vi "SVFA FFT Spectrum (Mag-Phase) (N Ch).vi"(0 "scaled signals [EU]":waveform(dbl)[](array[waveform]), 2 "window":T8=1 items=["None"=0, "Hanning"=1, "Hamming"=2, "Blackman-Harris"=3, "Exact Blackman"=4, "Blackman"=5, "Flat Top"=6, "4 Term B-Harris "=7, "7 Term B-Harris"=8, "Low Sidelobe"=9, "Force"=64, "Exponential"=65, "Blackman Nuttall"=11, "Triangle"=30, "Bartlett-Hanning"=31, "Bohman"=32, "Parzen"=33, "Welch"=34, "Kaiser"=60, "Dolph-Chebyshev"=61, "Gaussian"=62], 4 "view":T9={"dB On (T)"=TRUE, "unwrap phase (F)"=FALSE, "convert to degree (T)"=TRUE}, 5 "error in (no error)":errorcluster, 7 "averaging parameters":T7={"averaging mode"=enum."No averaging", "weighting mode"=enum."Exponential", "number of averages"=10, "linear mode"=enum."One shot"} {"number of averages" min=1 step=1}, 9 "restart averaging (F)":bool) -> (11 "averaging done":bool, 13 "averages completed":dbl, 14 "magnitudes [dB EU]":cluster{"f0":dbl, "df":dbl, "magnitude":dbl[]}[](array[cluster]) {"magnitude" format="%.2p"; "df" format="%.2p"; "f0" format="%.2p"}, 15 "magnitude unit labels":string[](array[string]), 16 "phases [degrees]":cluster{"f0":dbl, "df":dbl, "phase":dbl[]}[](array[cluster]) {"phase" format="%.2f"; "df" format="%.2f"; "f0" format="%.2f"}, 17 "phase unit labels":string[](array[string]), 18 "spectrum info":T1[](array[typedef]) {"x-axis units" items=["Time (s)"=0, "Frequency-CB (Hz)"=1, "Frequency-CPB (Hz)"=1248, "Frequency-Arbitrary (Hz)"=2357, "Quefrency (s)"=2, "Revolutions (rev)"=3, "Order"=4, "Speed (RPM)"=11, "Speed (rad/s)"=21, "Index"=65535]; "weighting filter" items=["Linear", "A-weighting", "B-weighting", "C-weighting", "ITU-R 468-4", "Dolby", "CCITT", "C-message", "Wb", "Wc", "Wd", "We", "Wf", "Wh", "Wj", "Wk", "Wm", "AES17 20 kHz lowpass", "AES17 40 kHz lowpass", "AES17 20 kHz highpass", "AES17 40 kHz highpass"]; "dB reference [EU]" format="%.2f"; "engineering units" items=["custom..."=0, "V"=1, "A"=21, "C"=30, "pC"=31, "s"=32, "-"=29, "Pa"=2, "N"=20, "g"=3, "m/s^2"=4, "m/s"=5, "m"=6, "mm/s"=12, "mm"=13, "micron/s"=14, "micron"=15, "in/s^2"=7, "in/s"=8, "in"=9, "mil/s"=10, "mil"=11, "rad/s^2"=16, "rad/s"=17, "rad"=18, "deg/s^2"=26, "deg/s"=27, "deg"=28, "RPM"=22, "cycle/s^2"=23, "Hz"=24, "cycle"=25, "strain"=19]; "spectral info"."window" items=["None "=0, "Hanning"=1, "Hamming"=2, "Blackman-Harris"=3, "Exact Blackman"=4, "Blackman"=5, "Flat Top"=6, "4 Term B-Harris "=7, "7 Term B-Harris"=8, "Low Sidelobe"=9, "Force - Exponential"=10, "Gaussian"=62]}, 19 "error out":errorcluster)   [LabVIEW 2017]
doc: "Computes the Fast Fourier Transform (FFT) spectrum of <B>scaled signal [EU]</B>. This VI returns FFT results as the magnitude and phase of the FFT spectrum. Wire data to the <B>scaled signal [EU]</B> input to determine the polymorphic instance to use or manually select the instance."
uses:
  <vilib>/addons/_NISVFA/_Shared subVIs/Controls/svc_Window.ctl
  <vilib>/addons/_NISVFA/_Shared subVIs/Controls/svc_Spectrum Info.ctl
  <vilib>/addons/_NISVFA/_Shared subVIs/Controls/svc_X-Axis Units.ctl
  <vilib>/addons/_NISVFA/_Shared subVIs/Controls/svc_Spectrum Type.ctl
  <vilib>/addons/_NISVFA/_Shared subVIs/Controls/svc_Engineering Units Text Ring.ctl
  <vilib>/addons/_NISVFA/_Shared subVIs/Controls/svc_Weighting Filter Text Ring.ctl
  <vilib>/addons/_NISVFA/_Shared subVIs/Controls/svc_Complimentary Spectrum Units.ctl
  <vilib>/Analysis/2dsp.llb/Real FFT.vi
  <vilib>/Analysis/2dsp.llb/Power Spectrum (DBL).vi
  <vilib>/addons/_NISVFA/_Shared subVIs/Windowing/svfa_Scaled Time Domain Window (1 Ch).vi
  <vilib>/addons/_NISVFA/_Shared subVIs/Spectrum Info/svfa_Build Spectrum Info.vi
  <vilib>/addons/_NISVFA/_Shared subVIs/Spectrum Averaging/svfa_No Average Array (complex).vi
  <vilib>/addons/_NISVFA/_Shared subVIs/Spectrum Averaging/svfa_Average Array (complex).vi
  <vilib>/addons/_NISVFA/_Shared subVIs/Spectrum Averaging/svfa_No Average Array (real).vi
  <vilib>/addons/_NISVFA/_Shared subVIs/Spectrum Averaging/svfa_Average Array (real).vi
  <vilib>/addons/_NISVFA/_Shared subVIs/Spectrum Averaging/svfa_Peak Hold Array.vi
  <vilib>/addons/_NISVFA/_Shared subVIs/Windowing/svfa_Scaled Time Domain Window (Array).vi
  <vilib>/addons/_NISVFA/_Shared subVIs/Common/svc_Get SV Channel Info.vi
  <vilib>/addons/_NISVFA/_Shared subVIs/Common/svc_Spectrum Units.vi
  <vilib>/Analysis/4window.llb/Force Window.vi
  <vilib>/Analysis/4window.llb/Force Window (DBL).vi
  <vilib>/Analysis/4window.llb/Exponential Window.vi
  <vilib>/Analysis/4window.llb/Exponential Window (DBL).vi
  <vilib>/Utility/error.llb/Error Cluster From Error Code.vi
  <vilib>/Analysis/0measdsp.llb/Scaled Time Domain Window.vi
  <vilib>/Analysis/0measdsp.llb/Scaled Time Domain Window (DBL).vi
  <vilib>/addons/_NISVFA/_Spectrum Processing/subVIs/svfa_Spectrum Info Window to windowTd Type Def.vi
  <vilib>/addons/_NISVFA/_Shared subVIs/Common/svc_Window Parameters.vi
  <vilib>/addons/_NISVFA/_Shared subVIs/Common/svc_Get Window Info.vi
  <vilib>/addons/_NISVFA/_Shared subVIs/Common/svc_Get Weighting Enum and Labels.vi
  <vilib>/addons/_NISVFA/_Shared subVIs/Common/svc_Unit Label Lexical Class.vi
  <vilib>/addons/_NISVFA/_Shared subVIs/Common/svc_Engineering Units to Unit Label.vi
  <vilib>/addons/_NISVFA/_Shared subVIs/Common/svc_Format Value (DBL).vi
  <vilib>/addons/_NISVFA/_Shared subVIs/Common/svc_Channel Info to Spectrum Info.vi
  <vilib>/addons/_NISVFA/_Shared subVIs/Common/svc_Unit Label to Engineering Units.vi
  <vilib>/Analysis/NI_AALPro.lvlib
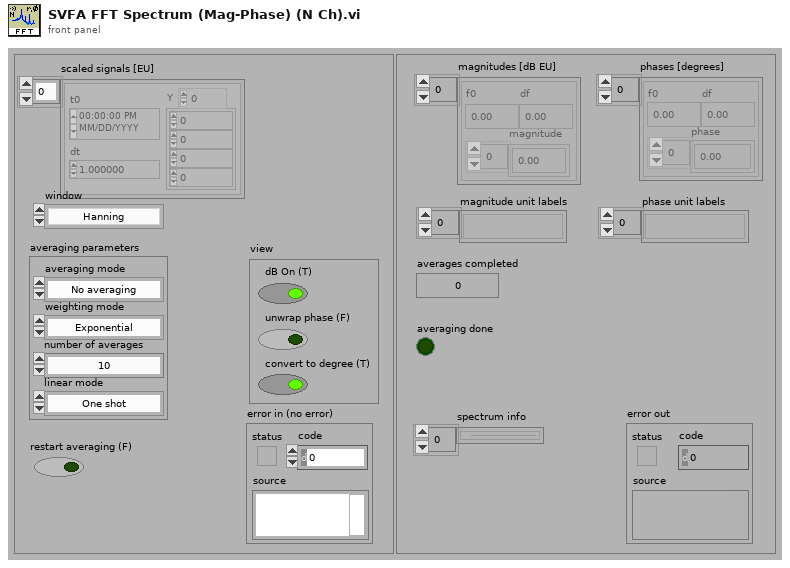
[diagram p1: front panel]
types:
  T1 = typedef "svc_Spectrum Info.ctl" = cluster{"channel name":string, "description":string, "x-axis units":T2, "spectral info":cluster{"spectrum type":T3, "linear/dB":enum16{"linear", "dB"}, "window":u16, "window size":i32, "FFT size":i32}, "engineering units":T4, "custom label":string, "dB reference [EU]":dbl, "peak units":enum16{"rms", "peak", "peak-peak"}, "weighting filter":T5, "spectral density?":bool, "unit label":string, "spectrum skewed?":bool, "complimentary spectrum units":T6}
  T2 = typedef "svc_X-Axis Units.ctl" = u16
  T3 = typedef "svc_Spectrum Type.ctl" = enum16{"FFT Spectrum [complex]", "Amplitude [Magnitude]", "Power [Magnitude^2]", "Cross Spectrum [complex]", "Frequency Response [Complex]"}
  T4 = typedef "svc_Engineering Units Text Ring.ctl" = u16
  T5 = typedef "svc_Weighting Filter Text Ring.ctl" = u16
  T6 = typedef "svc_Complimentary Spectrum Units.ctl" = enum16{"none", "radians", "degrees", "cycles", "imaginary"}
  T7 = cluster{"averaging mode":enum16{"No averaging", "Vector averaging", "RMS averaging", "Peak hold"}, "weighting mode":enum16{"Linear", "Exponential"}, "number of averages":u32, "linear mode":enum16{"One shot", "Auto restart"}}
  T8 = typedef "svc_Window.ctl" = u32
  T9 = cluster{"dB On (T)":bool, "unwrap phase (F)":bool, "convert to degree (T)":bool}
  T10 = cluster{"f0":dbl, "df":dbl, "complex spectrum":cdb[]}
  T11 = enum16{"Restart processing", "Continue processing", "Skip processing"}
  T12 = cluster{"complex FFT":cdb[], "real FFT":dbl[], "f0":dbl, "df":dbl, "averages completed":dbl, "averaging parameters":cluster{"averaging mode":enum16{"No averaging", "Vector averaging", "RMS averaging", "Peak hold"}, "weighting mode":enum16{"Linear", "Exponential"}, "number of averages":u32, "linear mode":enum16{"One shot", "Auto restart"}}}[]
  T13 = enum16{"No averaging", "Vector averaging", "RMS averaging", "Peak hold"}
  T14 = cluster{"complex FFT":cdb[], "real FFT":dbl[], "f0":dbl, "df":dbl, "averages completed":dbl, "averaging parameters":cluster{"averaging mode":enum16{"No averaging", "Vector averaging", "RMS averaging", "Peak hold"}, "weighting mode":enum16{"Linear", "Exponential"}, "number of averages":u32, "linear mode":enum16{"One shot", "Auto restart"}}}
  T15 = cluster{"complex FFT":cdb[], "Mag/Real FFT":dbl[], "f0":dbl, "df":dbl, "averages completed":dbl, "averaging parameters":cluster{"averaging mode":enum16{"No averaging", "Vector averaging", "RMS averaging", "Peak hold"}, "weighting mode":enum16{"Linear", "Exponential"}, "number of averages":u32, "linear mode":enum16{"One shot", "Auto restart"}}}
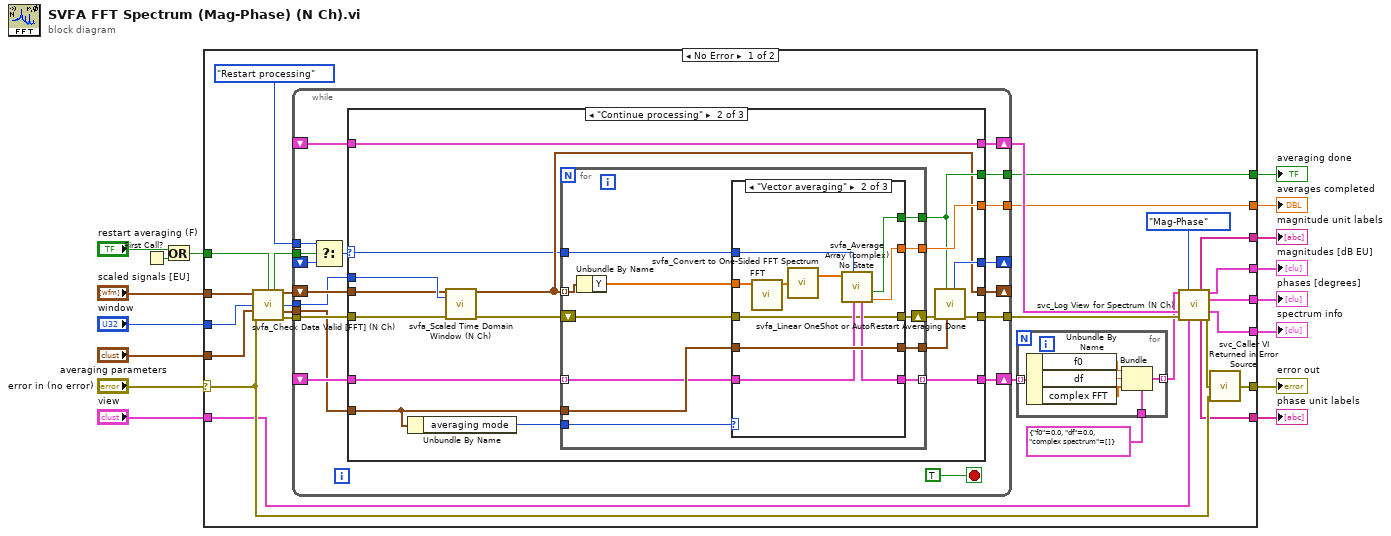
[diagram p0: block diagram]
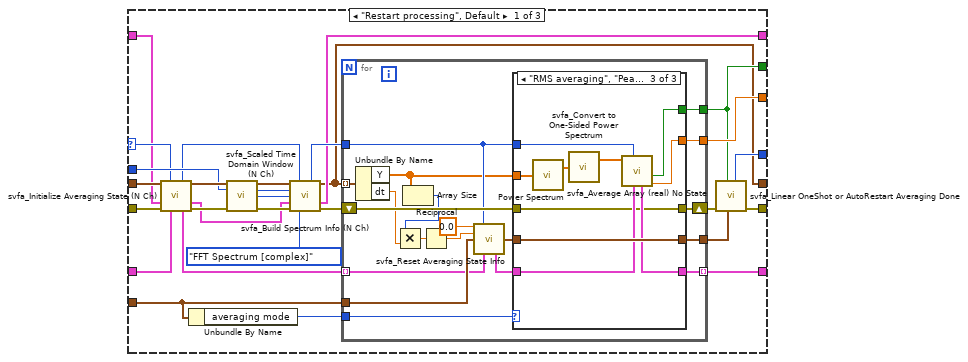
[diagram p2: hidden frame]
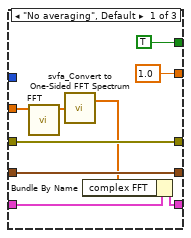
[diagram p3: hidden frame]
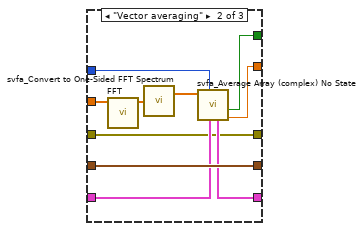
[diagram p4: hidden frame]
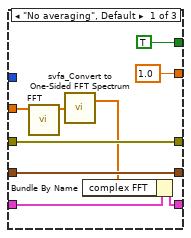
[diagram p5: hidden frame]
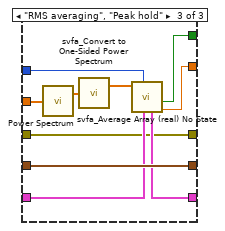
[diagram p6: hidden frame]
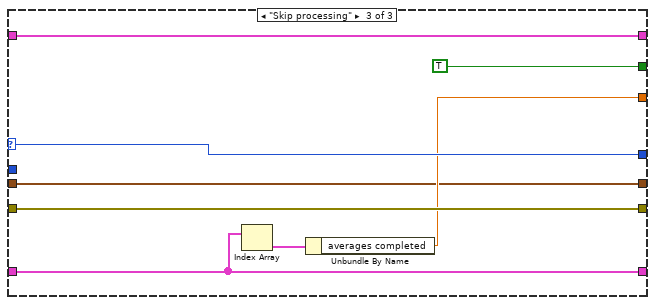
[diagram p7: hidden frame]
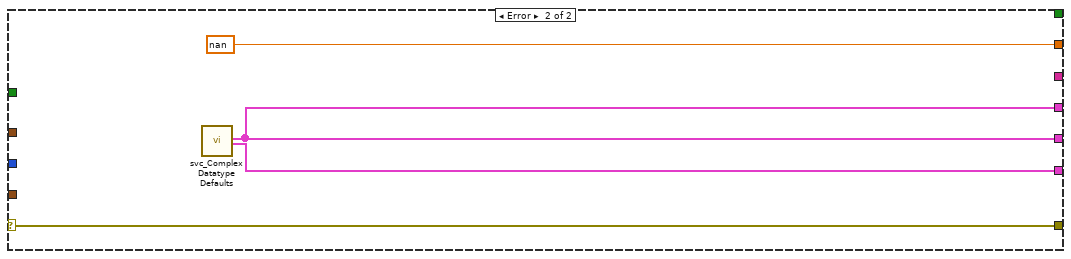
[diagram p8: hidden frame]
diagram:
  n1 = First Call?() -> (First Call?: T/F=w15:bool)
  n2 = Or(x="restart averaging (F)", y=w15) -> (x .or. y?=w10:bool)
  n3 = case shown="No Error" "error in (no error)" {
    selector: "error in (no error)" -> [w33 w213]
    tunnel: "scaled signals [EU]" -> [w43 _]
    tunnel: "averaging parameters" -> [w39 _]
    tunnel: w10 -> [w37 _]
    tunnel: [w34 w213] -> w3
    tunnel: [w42 w212] -> w6
    tunnel: [w23 _] -> w9
    tunnel: [w22 nan ("averages completed")] -> w8
    tunnel: [w40 w212] -> w5
    tunnel: [w36 _] -> w7
    tunnel: "window" -> [w38 _]
    tunnel: [w35 w211] -> w4
    tunnel: [w18 _] -> w2
    tunnel: "view" -> [w17 _]
    frame No Error {
      n4 = call <vilib>:"svfa_Check Data Valid [FFT] (N Ch).vi"("scaled signals"=w43, "restart averaging (F)"=w37, "window"=w38, "averaging parameters"=w39, "error in (no error)"=w33) -> ("restart averaging"=w30:bool, "dup scaled signals"=w26:waveform(dbl)[], "dup window"=w27:T8, "dup averaging parameters"=w28:T7, "error out"=w29:errorcluster)  [unwired: 6 in]
      n5 = while {
        tunnel: [w65] -> w22
        tunnel: [w61] -> w23
        tunnel: [w59] -> w24
        shift-left: _ -> [w62]
        shift-right: [w63] -> w21
        tunnel: w29 -> [w64]
        shift-right: [w57] -> w25
        shift-left: _ -> [w58]
        tunnel: w27 -> [w56]
        tunnel: w28 -> [w55]
        tunnel: T11."Restart processing" ("t") -> [w54]
        tunnel: w30 -> [w53]
        shift-right: [w60] -> _
        shift-left: _ -> [w52]
        shift-right: [w50] -> _
        shift-left: w26 -> [w66]
        stop <- TRUE stop-if-true
        n6 = Select(t=w54, s=w53, f=w52) -> (s? t:f=w51:T11)
        n7 = case shown="\"Continue processing\"" w51 {
          selector: w51 -> [w83 w148 w210]
          tunnel: w66 -> [w96 w150 w203]
          tunnel: [w94 w161 w206] -> w65
          tunnel: w64 -> [w74 w146 w209]
          tunnel: w56 -> [w91 w160 _]
          tunnel: w55 -> [w75 w152 _]
          tunnel: [w90 w159 w207] -> w63
          tunnel: w62 -> [w89 w147 w207]
          tunnel: [w87 w157 TRUE ("averaging done")] -> w61
          tunnel: [w86 w156 w210] -> w60
          tunnel: [w84 w154 w209] -> w59
          tunnel: w58 -> [w73 w151 w204]
          tunnel: [w71 w151 w204] -> w57
          tunnel: [w69 w149 w203] -> w50
          frame "Restart processing", Default {
            n8 = call <vilib>:"svfa_Initialize Averaging State (N Ch).vi"("Windowed Waveform(s)"=w96, "processing control in"=w83, "spectra info in"=w73, "error in (no error)"=w74, "state info"=w89) -> ("processing control out"=w70:T11, "Windowed Waveform(s)"=w93:waveform(dbl)[], "spectra info out"=w72:T1[], "state info"=w95:T12, "error out"=w92:errorcluster)  [unwired: 6 in]
            n9 = Unbundle By Name(w75) -> ("averaging mode"=w76:T13)
            n10 = call <vilib>:"svfa_Scaled Time Domain Window (N Ch).vi"("Scaled signal(s)"=w93, "window"=w91, "error in (no error)"=w92) -> ("Windowed Waveform(s)"=w82:waveform(dbl)[], "window"=w81:T8, "window length"=w68:i32, "error out"=w80:errorcluster)  [unwired: 8 in, 1 out]
            n11 = call <vilib>:"svfa_Build Spectrum Info (N Ch).vi"("scaled signal(s)"=w82, "processing control in"=w70, "window"=w81, "window size"=w68, "spectra info in"=w72, "error in (no error)"=w80, "spectrum type"=svc_Spectrum_Type."FFT Spectrum [complex]") -> ("dup processing control"=w78:T11, "dup scaled signals"=w69:waveform(dbl)[], "spectra info out"=w71:T1[], "error out"=w79:errorcluster)  [unwired: 5 in]
            n12 = for {
              tunnel: w78 -> [w106]
              tunnel: w95 -> [w101] mode=indexing
              tunnel: [w112] -> w87
              tunnel: [w114] -> w94
              tunnel: w69 -> [w108] mode=indexing
              tunnel: w75 -> [w103]
              tunnel: [w113] -> w90 mode=indexing
              tunnel: [w111] -> w88
              shift-right: [w115] -> w85
              shift-left: w79 -> [w109]
              tunnel: w76 -> [w110]
              n13 = Unbundle By Name ("Get Waveform Components")(w108) -> ("Y"=w98:dbl[], "dt"=w99:dbl)
              n14 = Array Size(array=w98) -> (size(s)=w97:i32)
              n15 = Multiply(x=w97, y=w99) -> (x*y=w107:dbl)
              n16 = Reciprocal(x=w107) -> (1/x=w104:dbl)
              n17 = call <vilib>:"svfa_Reset Averaging State Info.vi"("f0"=0.0, "processing control"=w106, "df"=w104, "averaging parameters"=w103, "averaging state info in"=w101) -> ("dup averaging parameters"=w102:T7, "averaging state info out"=w100:T14)  [unwired: 9 in]
              n18 = case shown="\"RMS averaging\", \"Peak hold\"" w110 {
                tunnel: w106 -> [_ w130 w140]
                tunnel: w100 -> [w120 w127 w139]
                tunnel: w98 -> [w117 w133 w143]
                tunnel: [w121 w125 w135] -> w115
                tunnel: [TRUE ("averaging done") w129 w137] -> w112
                tunnel: [1.0 ("averages completed") w128 w136] -> w114
                tunnel: w109 -> [w121 w125 w135]
                tunnel: w102 -> [w122 w131 w141]
                tunnel: [w119 w126 w138] -> w113
                tunnel: [w122 w131 w141] -> w111
                frame "No averaging", Default {
                  n19 = call-poly <vilib>:"FFT.vi"("X"=w117) -> ("FFT {X}"=w118:cdb[])  [unwired: 9 in, 1 out]
                  n20 = call <vilib>:"svfa_Convert to One-Sided FFT Spectrum.vi"("two-sided FFT spectrum"=w118) -> ("one-sided FFT spectrum"=w116:cdb[])  [unwired: 1 out]
                  n21 = Bundle By Name(cluster=w120, "complex FFT"=w116) -> (w119:T14)
                }
                frame "Vector averaging" {
                  n22 = call-poly <vilib>:"FFT.vi"("X"=w133) -> ("FFT {X}"=w134:cdb[])  [unwired: 9 in, 1 out]
                  n23 = call <vilib>:"svfa_Convert to One-Sided FFT Spectrum.vi"("two-sided FFT spectrum"=w134) -> ("one-sided FFT spectrum"=w132:cdb[])  [unwired: 1 out]
                  n24 = call <vilib>:"svfa_Average Array (complex) No State.vi"("averaging state info in"=w127, "processing control"=w130, "array"=w132) -> ("averages completed"=w128:dbl, "averaging done"=w129:bool, "averaging state info out"=w126:T15)  [unwired: 5 in, 1 out]
                }
                frame "RMS averaging", "Peak hold" {
                  n25 = call-poly <vilib>:"Power Spectrum.vi"("X"=w143) -> ("Power Spectrum"=w144:dbl[])  [unwired: 1 out]
                  n26 = call <vilib>:"svfa_Convert to One-Sided Power Spectrum.vi"("two-sided power spectrum"=w144) -> ("one-sided power spectrum"=w142:dbl[])  [unwired: 1 out]
                  n27 = call <vilib>:"svfa_Average Array (real) No State.vi"("averaging state info in"=w139, "processing control"=w140, "array"=w142) -> ("averages completed"=w136:dbl, "averaging done"=w137:bool, "averaging state info out"=w138:T15)  [unwired: 5 in, 1 out]
                }
              }
            }
            n28 = call <vilib>:"svfa_Linear OneShot or AutoRestart Averaging Done.vi"("averaging parameters"=w88, "averaging done"=w87, "error in (no error)"=w85) -> ("error out"=w84:errorcluster, "processing control"=w86:T11)  [unwired: 7 in]
          }
          frame "Continue processing" {
            n29 = Unbundle By Name(w152) -> ("averaging mode"=w153:T13)
            n30 = call <vilib>:"svfa_Scaled Time Domain Window (N Ch).vi"("Scaled signal(s)"=w150, "window"=w160, "error in (no error)"=w146) -> ("Windowed Waveform(s)"=w149:waveform(dbl)[], "error out"=w145:errorcluster)  [unwired: 8 in, 3 out]
            n31 = for {
              tunnel: w148 -> [w164]
              tunnel: w147 -> [w162] mode=indexing
              tunnel: [w170] -> w157
              tunnel: [w172] -> w161
              tunnel: w149 -> [w166] mode=indexing
              tunnel: w152 -> [w163]
              tunnel: [w171] -> w159 mode=indexing
              tunnel: [w169] -> w158
              shift-right: [w173] -> w155
              shift-left: w145 -> [w167]
              tunnel: w153 -> [w168]
              n32 = Unbundle By Name ("Get Waveform Components")(w166) -> ("Y"=w165:dbl[])
              n33 = case shown="\"Vector averaging\"" w168 {
                tunnel: w164 -> [_ w188 w198]
                tunnel: w162 -> [w178 w185 w197]
                tunnel: w165 -> [w175 w191 w201]
                tunnel: [w179 w183 w193] -> w173
                tunnel: [TRUE ("averaging done") w187 w195] -> w170
                tunnel: [1.0 ("averages completed") w186 w194] -> w172
                tunnel: w167 -> [w179 w183 w193]
                tunnel: w163 -> [w180 w189 w199]
                tunnel: [w177 w184 w196] -> w171
                tunnel: [w180 w189 w199] -> w169
                frame "No averaging", Default {
                  n34 = call-poly <vilib>:"FFT.vi"("X"=w175) -> ("FFT {X}"=w176:cdb[])  [unwired: 9 in, 1 out]
                  n35 = call <vilib>:"svfa_Convert to One-Sided FFT Spectrum.vi"("two-sided FFT spectrum"=w176) -> ("one-sided FFT spectrum"=w174:cdb[])  [unwired: 1 out]
                  n36 = Bundle By Name(cluster=w178, "complex FFT"=w174) -> (w177:T15)
                }
                frame "Vector averaging" {
                  n37 = call-poly <vilib>:"FFT.vi"("X"=w191) -> ("FFT {X}"=w192:cdb[])  [unwired: 9 in, 1 out]
                  n38 = call <vilib>:"svfa_Convert to One-Sided FFT Spectrum.vi"("two-sided FFT spectrum"=w192) -> ("one-sided FFT spectrum"=w190:cdb[])  [unwired: 1 out]
                  n39 = call <vilib>:"svfa_Average Array (complex) No State.vi"("averaging state info in"=w185, "processing control"=w188, "array"=w190) -> ("averages completed"=w186:dbl, "averaging done"=w187:bool, "averaging state info out"=w184:T15)  [unwired: 5 in, 1 out]
                }
                frame "RMS averaging", "Peak hold" {
                  n40 = call-poly <vilib>:"Power Spectrum.vi"("X"=w201) -> ("Power Spectrum"=w202:dbl[])  [unwired: 1 out]
                  n41 = call <vilib>:"svfa_Convert to One-Sided Power Spectrum.vi"("two-sided power spectrum"=w202) -> ("one-sided power spectrum"=w200:dbl[])  [unwired: 1 out]
                  n42 = call <vilib>:"svfa_Average Array (real) No State.vi"("averaging state info in"=w197, "processing control"=w198, "array"=w200) -> ("averages completed"=w194:dbl, "averaging done"=w195:bool, "averaging state info out"=w196:T15)  [unwired: 5 in, 1 out]
                }
              }
            }
            n43 = call <vilib>:"svfa_Linear OneShot or AutoRestart Averaging Done.vi"("averaging parameters"=w158, "averaging done"=w157, "error in (no error)"=w155) -> ("error out"=w154:errorcluster, "processing control"=w156:T11)  [unwired: 7 in]
          }
          frame "Skip processing" {
            n44 = Index Array(array=w207) -> (element=w205:T15)  [unwired: 1 in]
            n45 = Unbundle By Name(w205) -> ("averages completed"=w206:dbl)
          }
        }
      }
      n46 = for {
        tunnel: w21 -> [w49] mode=indexing
        tunnel: T10 {"f0"=0.0, "df"=0.0, "complex spectrum"=[]} ("cluster") -> [w48]
        tunnel: [w44] -> w19 mode=indexing
        n47 = Unbundle By Name(w49) -> ("f0"=w46:dbl, "df"=w47:dbl, "complex FFT"=w45:cdb[])
        n48 = Bundle(cluster=w48, "f0"=w46, "df"=w47, "complex spectrum"=w45) -> (w44:T10)
      }
      n49 = call <vilib>:"svc_Log View for Spectrum (N Ch).vi"("complex spectra"=w19, "View"=enum16{"Mag-Phase", "Real-Imaginary"}."Mag-Phase", "spectra info in"=w25, "error in (no error)"=w24, "view"=w17) -> ("unit label [mag or real]"=w36:string[], "magnitude or real"=w42:cluster{"f0":dbl, "df":dbl, "magnitude":dbl[]}[], "phase or imaginary"=w40:cluster{"f0":dbl, "df":dbl, "magnitude":dbl[]}[], "spectra info out"=w35:T1[], "unit label [phase or imag]"=w18:string[], "error out"=w41:errorcluster)  [unwired: 5 in]
      n50 = call <vilib>:"svc_Caller VI Returned in Error Source.vi"("warning input to caller"=w33, "error in (no error)"=w41) -> ("error out"=w34:errorcluster)  [unwired: 3 in]
    }
    frame Error {
      n51 = call <vilib>:"svc_Complex Datatype Defaults.vi"() -> ("empty array of spectra"=w212:cluster{"f0":dbl, "df":dbl, "magnitude":dbl[]}[], "empty array of spectrum info"=w211:T1[])  [unwired: 11 in, 7 out]
    }
  }
  "error out" <- w3
  "averaging done" <- w9
  "averages completed" <- w8
  "magnitude unit labels" <- w7
  "magnitudes [dB EU]" <- w6
  "phases [degrees]" <- w5
  "phase unit labels" <- w2
  "spectrum info" <- w4
